vi "Q Driver.vi"(0 "Q Name":string, 5 "State In":string, 7 "States s[]":string[](array[string]), 11 "error in (no error)":errorcluster, 13 "Q Operation":T1) -> (4 "State Out":string, 15 "error out":errorcluster)   [LabVIEW 2020, in "I2C Controller Lib.lvlib"]
uses:
  I2C Controller Lib.lvlib
  TypeDef/Queue Operation Mode.ctl
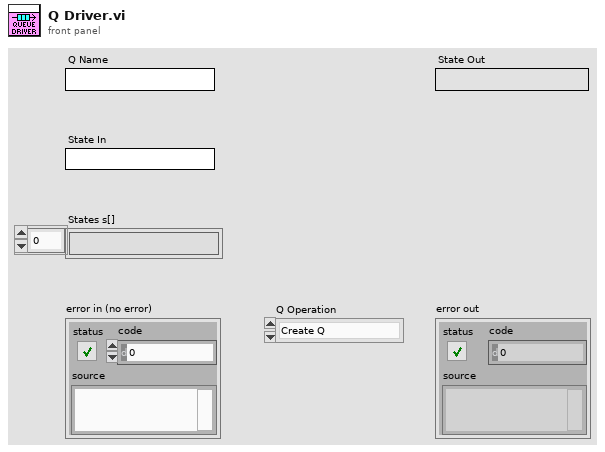
[diagram p1: front panel]
types:
  T1 = typedef "I2C Controller Lib.lvlib/Queue Operation Mode.ctl" = enum16{"Create Q", "Enqueue", "Enqueue N", "Enstack", "Dequeue", "Flush Q", "Close Q"}
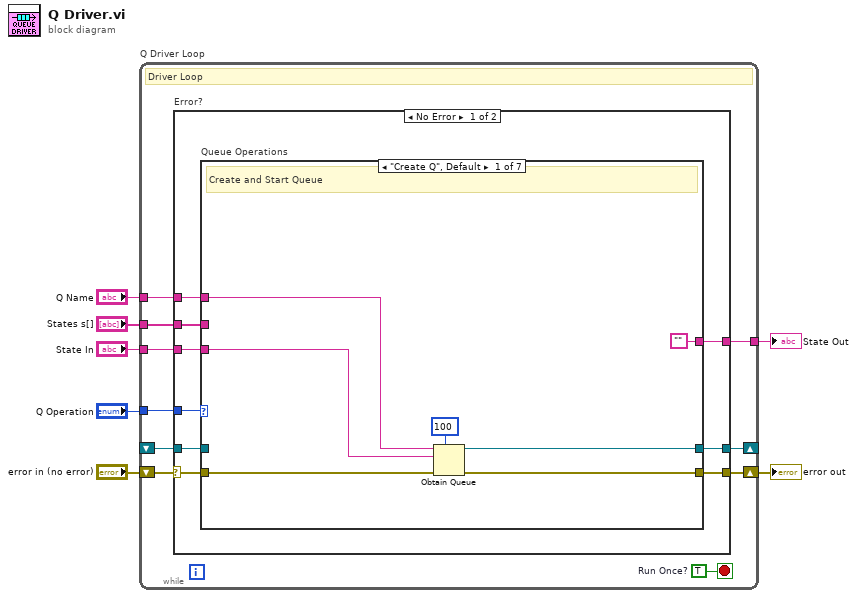
[diagram p0: block diagram]
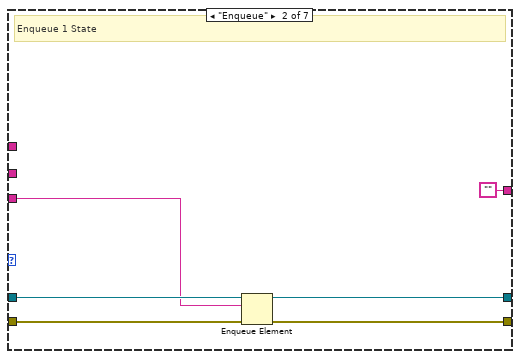
[diagram p2: hidden frame]
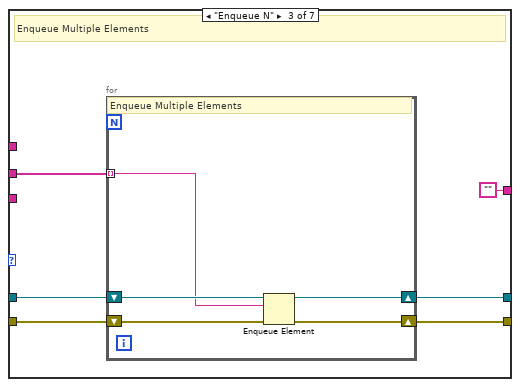
[diagram p3: hidden frame]
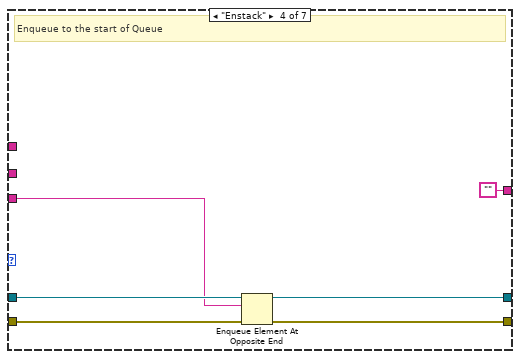
[diagram p4: hidden frame]
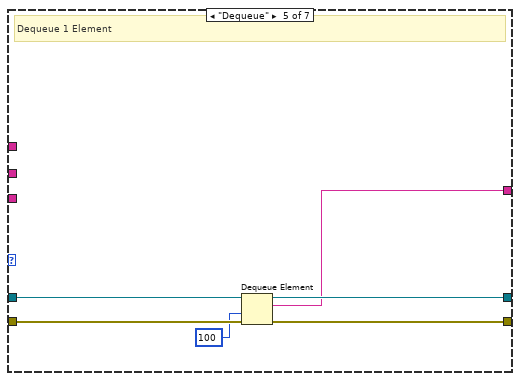
[diagram p5: hidden frame]
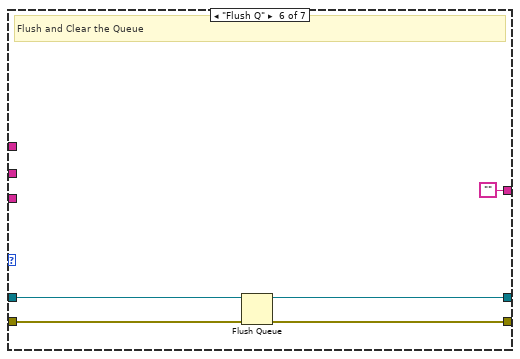
[diagram p6: hidden frame]
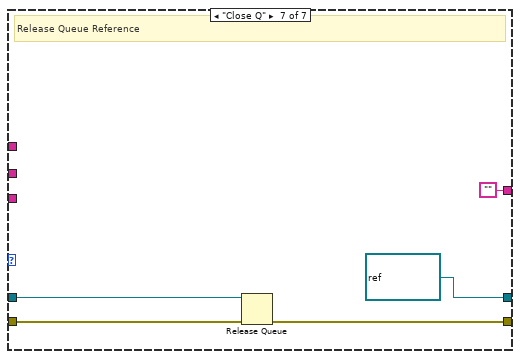
[diagram p7: hidden frame]
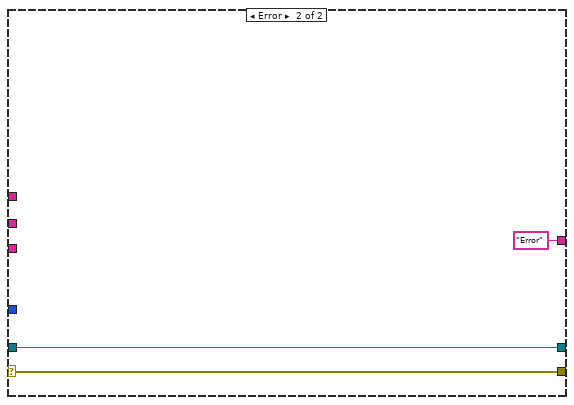
[diagram p8: hidden frame]
diagram:
  n1 = while "Q Driver Loop" {
    tunnel: "Q Operation" -> [w8]
    shift-right: [w15] -> _
    shift-left: _ -> [w14]
    tunnel: "States s[]" -> [w13]
    tunnel: "State In" -> [w12]
    tunnel: "Q Name" -> [w11]
    shift-right: [w16] -> w6
    shift-left: "error in (no error)" -> [w17]
    tunnel: [w10] -> w2
    stop <- w9 stop-if-true
    w9 = TRUE  # Run Once?
    # "Driver Loop"
    n2 = case "Error?" shown="No Error" w17 {
      selector: w17 -> [w25 w75]
      tunnel: [w26 w75] -> w16
      tunnel: w8 -> [w24 _]
      tunnel: [w23 w74] -> w15
      tunnel: w14 -> [w22 w74]
      tunnel: w13 -> [w21 _]
      tunnel: w12 -> [w20 _]
      tunnel: w11 -> [w19 _]
      tunnel: [w18 "Error"] -> w10
      frame No Error {
        n3 = case "Queue Operations" shown="\"Create Q\", Default" w24 {
          tunnel: [w32 w38 w45 w55 w61 w66 w71] -> w26
          tunnel: w25 -> [w33 w39 w44 w56 w62 w67 w72]
          tunnel: [w31 w36 w43 w52 w58 w64 refnum<queue> refnum ("queue out")] -> w23
          tunnel: w22 -> [_ w37 w42 w54 w60 w65 w70]
          tunnel: w21 -> [_ _ w41 _ _ _ _]
          tunnel: w20 -> [w28 w35 _ w53 _ _ _]
          tunnel: w19 -> [w30 _ _ _ _ _ _]
          tunnel: ["" ("Empty String Constant") "" ("Empty String Constant") "" ("Empty String Constant") "" ("Empty String Constant") w57 "" ("Empty String Constant") "" ("Empty String Constant")] -> w18
          frame "Create Q", Default {
            # "Create and Start Queue"
            n4 = Obtain Queue(max queue size (-1, unlimited)=100, name (unnamed)=w30, element data type=w28, error in (no error)=w33) -> (queue out=w31:refnum<queue>, error out=w32:errorcluster)  [unwired: 1 in, 1 out]
          }
          frame "Enqueue" {
            # "Enqueue 1 State"
            n5 = Enqueue Element(queue=w37, element=w35, error in (no error)=w39) -> (queue out=w36:refnum<queue>, error out=w38:errorcluster)  [unwired: 1 in, 1 out]
          }
          frame "Enqueue N" {
            # "Enqueue Multiple Elements"
            n6 = for {
              tunnel: w41 -> [w46] mode=indexing
              shift-right: [w49] -> w45
              shift-left: w44 -> [w50]
              shift-right: [w48] -> w43
              shift-left: w42 -> [w47]
              # "Enqueue Multiple Elements"
              n7 = Enqueue Element(queue=w47, element=w46, error in (no error)=w50) -> (queue out=w48:refnum<queue>, error out=w49:errorcluster)  [unwired: 1 in, 1 out]
            }
          }
          frame "Enstack" {
            # "Enqueue to the start of Queue"
            n8 = Enqueue Element At Opposite End(queue=w54, element=w53, error in (no error)=w56) -> (queue out=w52:refnum<queue>, error out=w55:errorcluster)  [unwired: 1 in, 1 out]
          }
          frame "Dequeue" {
            # "Dequeue 1 Element"
            n9 = Dequeue Element(queue=w60, timeout in ms (-1)=100, error in (no error)=w62) -> (queue out=w58:refnum<queue>, element=w57:string, error out=w61:errorcluster)  [unwired: 1 out]
          }
          frame "Flush Q" {
            # "Flush and Clear the Queue"
            n10 = Flush Queue(queue=w65, error in (no error)=w67) -> (queue out=w64:refnum<queue>, error out=w66:errorcluster)  [unwired: 1 out]
          }
          frame "Close Q" {
            # "Release Queue Reference"
            n11 = Release Queue(queue=w70, error in (no error)=w72) -> (error out=w71:errorcluster)  [unwired: 1 in, 2 out]
          }
        }
      }
      frame Error {
      }
    }
  }
  "error out" <- w6
  "State Out" <- w2
